vi "main.vi"() -> ()   [LabVIEW 2022 SP3]
uses:
  <vilib>/addons/Modulation/niDMT.lvlib
  <vilib>/addons/Modulation/niAMT.lvlib
  <vilib>/addons/Modulation/Digital/General/MT Format Eye Diagram (complex).vi
panel:
  out "constelation 2":T1(graph)
  out "graph 2":dbl[](graph)
  out "Constelation":T1(graph)
  out "graph 1":dbl[][](graph)
  out "symbols out":cdb[](array[numeric]) format="%.2f"
  in  "input bit stream":i8[](array[numeric])
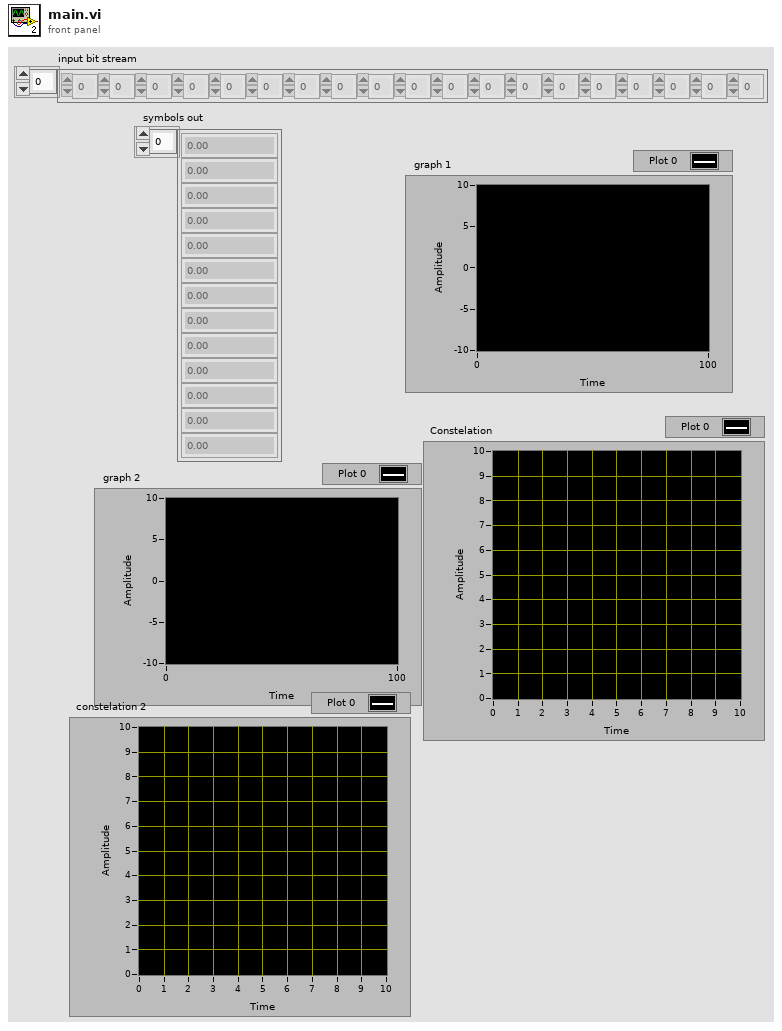
[diagram p1: front panel]
types:
  T1 = cluster{"constellation":dbl[], "oversampled data":dbl[]}[]
  T2 = typedef "niAMT.lvlib/Complex Data Waveform.ctl" = cluster{"t0":dbl, "dt":dbl, "Y":cdb[]}
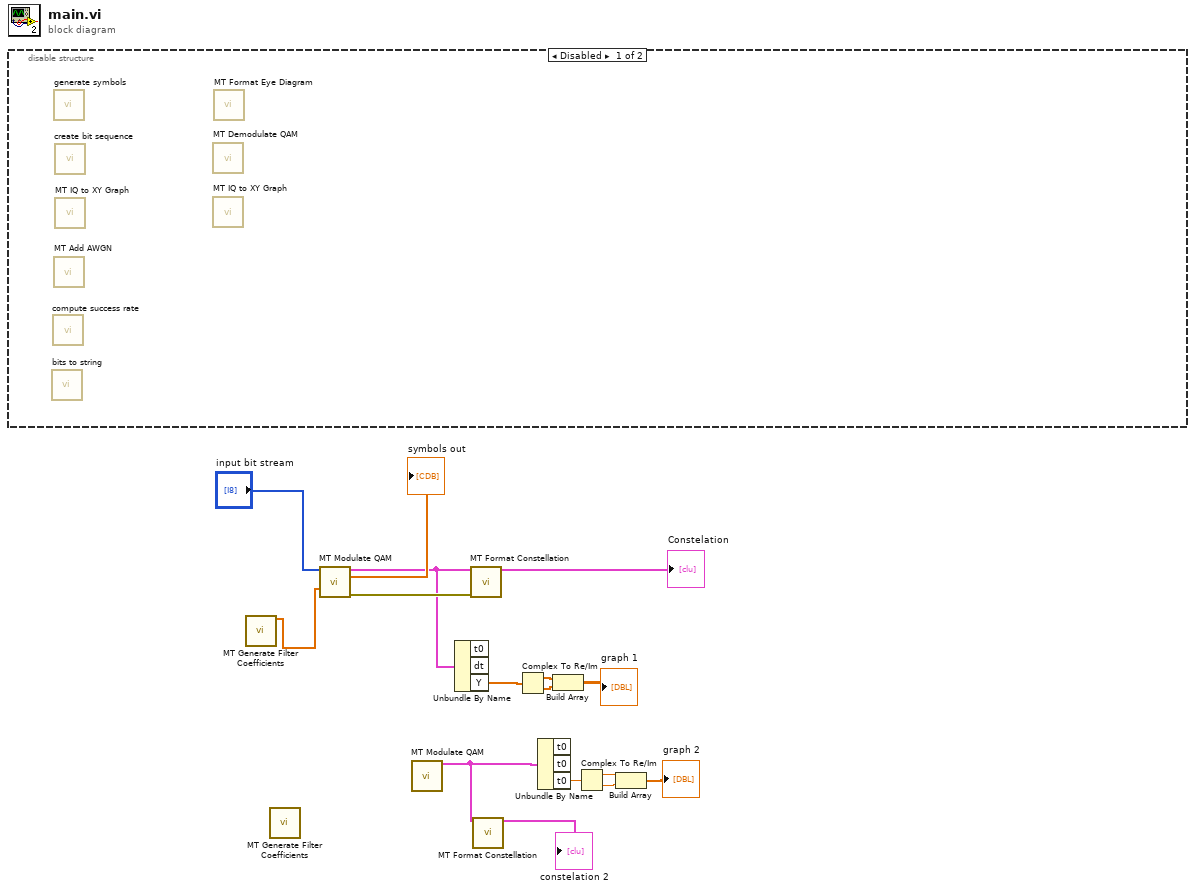
[diagram p0: block diagram]
diagram:
  n1 = disable-structure shown="Disabled" {
    frame Disabled {
      n2 = call "bits to string.vi"() -> ()  [unwired: 11 in, 1 out]
      n3 = call "compute success rate.vi"() -> ()  [unwired: 11 in, 1 out]
      n4 = call "generate symbols.vi"() -> ()  [unwired: 11 in, 1 out]
      n5 = call <vilib>:"MT Add AWGN.vi"() -> ()  [unwired: 13 in, 3 out]
      n6 = call "create bit sequence.vi"() -> ()  [unwired: 10 in, 2 out]
      n7 = call <vilib>:"MT IQ to XY Graph.vi"() -> ()  [unwired: 13 in, 3 out]
      n8 = call <vilib>:"MT Demodulate QAM.vi"() -> ()  [unwired: 11 in, 5 out]
      n9 = call <vilib>:"MT IQ to XY Graph.vi"() -> ()  [unwired: 13 in, 3 out]
      n10 = call-poly <vilib>:"MT Format Eye Diagram.vi"() -> ()  [unwired: 14 in, 2 out]
    }
    frame Enabled {
    }
  }
  n11 = call <vilib>:"MT Generate Filter Coefficients.vi"() -> ("pulse shaping filter coefficients"=w14:dbl[])  [unwired: 13 in, 2 out]
  n12 = call <vilib>:"MT Generate Filter Coefficients.vi"() -> ()  [unwired: 13 in, 3 out]
  n13 = call <vilib>:"MT Modulate QAM.vi"("input bit stream"="input bit stream", "pulse shaping filter coefficients"=w14) -> ("output complex waveform"=w11:T2, "symbols out"=→"symbols out":cdb[], "error out"=w15:errorcluster)  [unwired: 11 in]
  n14 = call <vilib>:"MT Modulate QAM.vi"() -> ("output complex waveform"=w2:T2)  [unwired: 13 in, 2 out]
  n15 = Unbundle By Name(w11) -> ("Y"=w10:cdb[])  [unwired: 2 out]
  n16 = call <vilib>:"MT Format Constellation.vi"("waveform"=w11, "error in (no error)"=w15) -> ("constellation graph"=→"Constelation":T1)  [unwired: 12 in, 1 out]
  n17 = call <vilib>:"MT Format Constellation.vi"("waveform"=w2) -> ("constellation graph"=→"constelation 2":T1)  [unwired: 13 in, 1 out]
  n18 = Complex To Re/Im(x + iy=w10) -> (x=w9:dbl[], y=w8:dbl[])
  n19 = Unbundle By Name(w2) -> ("t0"=w6:dbl)  [unwired: 2 out]
  n20 = Build Array(w9, w8) -> (→"graph 1":dbl[][])
  n21 = Complex To Re/Im(x + iy=w6) -> (x=w5:dbl, y=w4:dbl)
  n22 = Build Array(w5, w4) -> (→"graph 2":dbl[])
